vi "Charging_Enable Output.vi"(8 "error in (no error)":errorcluster, 10 "enable output (true)":bool=TRUE caption="channel enabled (True)", 11 "instrument handle":refnum<k15>) -> (0 "error out":errorcluster, 3 "instrument handle out":refnum<k15>)   [LabVIEW 2010]
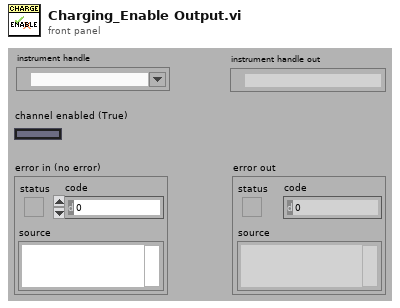
[diagram p1: front panel]
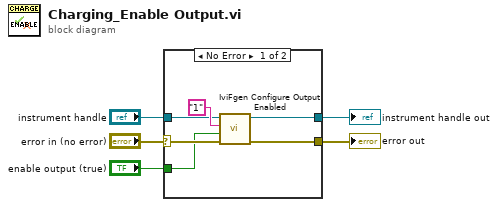
[diagram p0: block diagram]
diagram:
  n1 = case shown="No Error" "error in (no error)" {
    selector: "error in (no error)" -> [w10 w12]
    tunnel: [w9 w12] -> w4
    tunnel: "enable output (true)" -> [w8 _]
    tunnel: "instrument handle" -> [w7 w13]
    tunnel: [w6 w13] -> w1
    frame No Error {
      n2 = call <vilib>:"IviFgen Configure Output Enabled.vi"("error in (no error)"=w10, "channel enabled (True)"=w8, "channel name (\"CHANNEL1\")"="1" ("channel name (\"CHANNEL1\")"), "instrument handle"=w7) -> ("error out"=w9:errorcluster, "instrument handle out"=w6:refnum<k15>)  [unwired: 6 in]
    }
    frame Error {
    }
  }
  "error out" <- w4
  "instrument handle out" <- w1
